vi "Remove Self Index from Indexes.vi"(9 "Self index in":i32, 10 "Indexes in":i32[](array[numeric])) -> (1 "Found?":bool, 2 "Indexes out":i32[](array[numeric]))   [LabVIEW 2024, in "AI Manager.lvclass"]
doc: "MIT Licence\nCopyright (c) 2024 David Grollier"
uses:
  AI Manager.lvclass
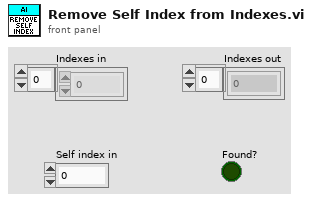
[diagram p1: front panel]
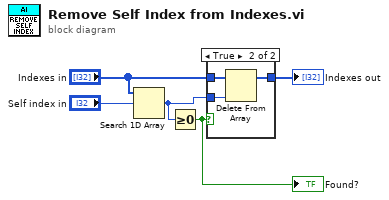
[diagram p0: block diagram]
diagram:
  n1 = Search 1D Array(1D array="Indexes in", element="Self index in") -> (index of element=w1:i32)  [unwired: 1 in]
  n2 = Greater Or Equal To 0?(x=w1) -> (x >= 0?=w3:bool)
  "Found?" <- w3
  n3 = case shown="True" w3 {
    tunnel: "Indexes in" -> [w6 w9]
    tunnel: [w6 w8] -> w5
    tunnel: w1 -> [_ w7]
    frame False {
    }
    frame True {
      n4 = Delete From Array(array=w9, index=w7) -> (array with subset deleted=w8:i32[])  [unwired: 1 in, 1 out]
    }
  }
  "Indexes out" <- w5
